vi "ICM aDBL.vi"(9 "Reverse Bytes":bool, 10 "Swap Bytes":bool, 11 "String In":string) -> (1 "Value DBL":dbl, 2 "Value":dbl, 3 "String Out":string)   [LabVIEW 2015]
doc: "ICM aDBL.vi\n\n This VI is used to parse binary data that contains a Double Precision Real.\n\nThis VI was original part of the OSDS system.\n\nInstrument Communication Module Version 1.0\nSeptember, 2017 Original Code Consulting David Thomson\n www.originalcode.com"
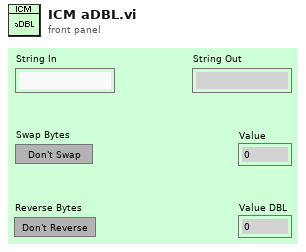
[diagram p1: front panel]
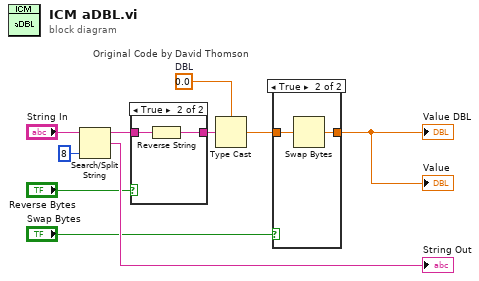
[diagram p0: block diagram]
diagram:
  w8 = 0.0  # DBL
  n1 = Search/Split String(string="String In", offset (0)=8) -> (substring before match=w6:string, match + rest of string=→"String Out":string)  [unwired: 2 out]
  n2 = case "Original Code by David Thomson" shown="True" "Reverse Bytes" {
    tunnel: w6 -> [w11 w13]
    tunnel: [w11 w12] -> w5
    frame False {
    }
    frame True {
      n3 = Reverse String(1:w13) -> (0:w12:string)
    }
  }
  n4 = Type Cast(type=w8, x=w5) -> (*(type *) &x=w3:dbl)
  n5 = case shown="True" "Swap Bytes" {
    tunnel: w3 -> [w14 w16]
    tunnel: [w14 w15] -> w2
    frame False {
    }
    frame True {
      n6 = Swap Bytes(anything=w16) -> (byte swapped=w15:dbl)
    }
  }
  "Value" <- w2
  "Value DBL" <- w2
